vi "GPS Input format.vi"(1 "Input":string) -> (0 "Output":string)   [LabVIEW 2016]
panel:
  # "Formats the input command into correct NMEA input."
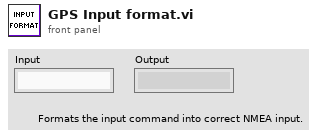
[diagram p1: front panel]
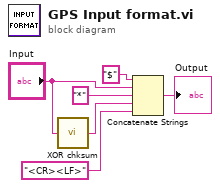
[diagram p0: block diagram]
diagram:
  n1 = call "XOR chksum.vi"("String"="Input") -> ("Checksum"=w2:string)
  n2 = Concatenate Strings("$" ("string"), "Input", "*" ("string"), w2, "<CR><LF>" ("string")) -> (→"Output":string)
